vi "Spline Interpolation 1D.vi"(4 "final boundary":T1, 6 "initial boundary":T1, 9 "xi":dbl[](array[numeric]) format="%_6g", 10 "X":dbl[](array[numeric]), 11 "Y":dbl[](array[numeric])) -> (0 "error":i32, 1 "piecewise polynomial":T2 {"x locations" format="%.4g"; "coefficients" format="%.4g"}, 3 "yi":dbl[](array[numeric]) format="%_6g")   [LabVIEW 2017, in "NI_Gmath.lvlib"]
doc: "Performs one-dimensional interpolation using the spline interpolation method based on the lookup table defined by <B>X</B> and <B>Y</B>."
uses:
  <vilib>/gmath/NI_Gmath.lvlib
  <vilib>/gmath/interp.llb/in_piecewise interp poly control.ctl
  <vilib>/Analysis/7linalg.llb/Solve Linear Equations (single right hand).vi
  <vilib>/Analysis/baseanly.llb/Solve Linear Equations By Cholesky.vi
  <vilib>/Analysis/baseanly.llb/Real Matrix to Compact Array.vi
  <vilib>/Analysis/baseanly.llb/Real Compact Tri-Matrix Linear Eqs.vi
  <vilib>/Analysis/7linalg.llb/Solve Linear Eqs (General).vi
  <vilib>/Analysis/7linalg.llb/Solve Linear Eqs (Gen, single right hand).vi
  <vilib>/Analysis/NI_AALPro.lvlib
panel:
  # "Spline Interpolation 1D"
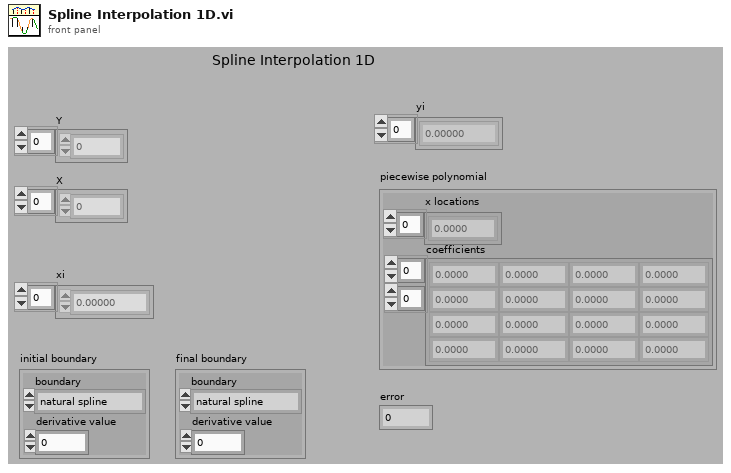
[diagram p1: front panel]
types:
  T1 = cluster{"boundary":enum16{"natural spline", "not-a-knot", "1st derivative", "2nd derivative"}, "derivative value":dbl}
  T2 = typedef "NI_Gmath.lvlib/in_piecewise interp poly control.ctl" = cluster{"x locations":dbl[], "coefficients":dbl[][]}
  T3 = typedef "NI_Matrix.lvlib/RealMatrix.ctl" = dbl[][]
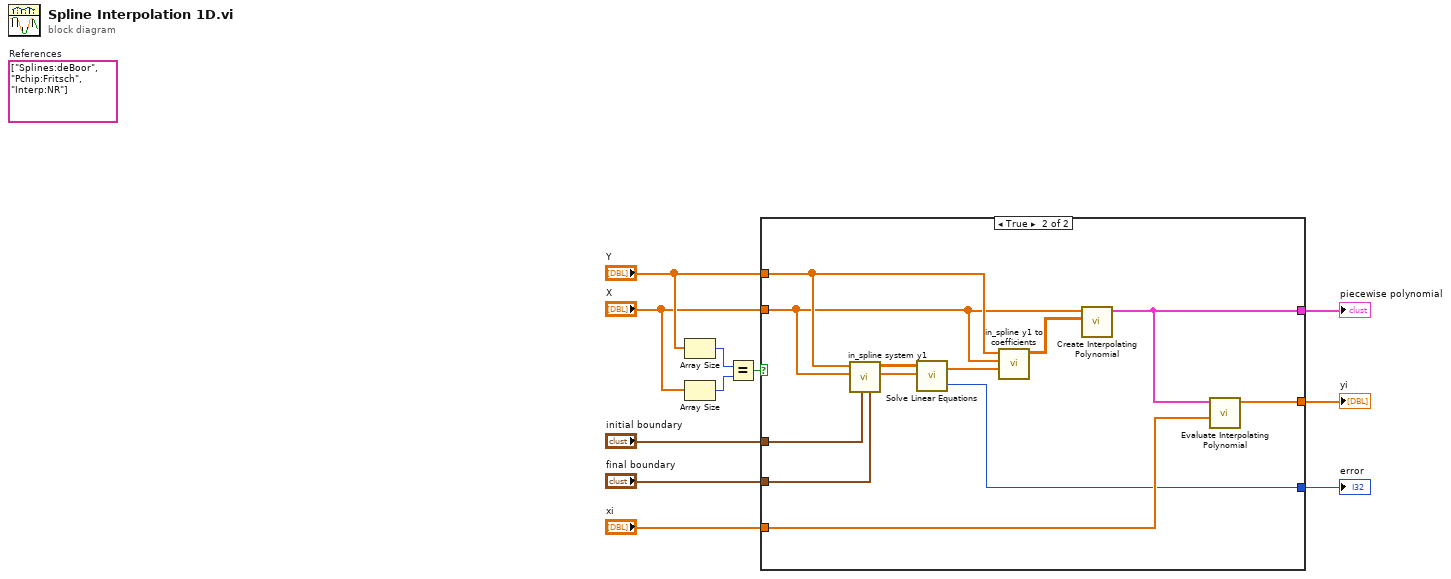
[diagram p0: block diagram]
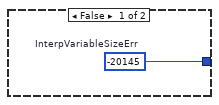
[diagram p2: hidden frame]
diagram:
  (unwired) string[] ["Splines:deBoor", "Pchip:Fritsch", "Interp:NR"]  # References
  n1 = Array Size(array="Y") -> (size(s)=w11:i32)
  n2 = Array Size(array="X") -> (size(s)=w10:i32)
  n3 = Equal?(x=w11, y=w10) -> (x = y?=w7:bool)
  n4 = case shown="True" w7 {
    tunnel: "Y" -> [_ w21]
    tunnel: "X" -> [_ w15]
    tunnel: [w12 w13] -> w6
    tunnel: "initial boundary" -> [_ w20]
    tunnel: "final boundary" -> [_ w19]
    tunnel: "xi" -> [_ w18]
    tunnel: [_ w17] -> w2
    tunnel: [_ w14] -> w1
    frame False {
      w12 = -20145  # InterpVariableSizeErr
    }
    frame True {
      n5 = call <vilib>:"in_spline system y1.vi"("final boundary"=w19, "initial boundary"=w20, "X"=w15, "Y"=w21) -> ("b"=w23:dbl[], "A"=w24:T3)  [unwired: 6 in]
      n6 = call-poly <vilib>:"Solve Linear Equations.vi"("Known Vector"=w23, "Input Matrix"=w24) -> ("error"=w13:i32, "Solution Vector"=w22:dbl[])  [unwired: 1 in]
      n7 = call <vilib>:"in_spline y1 to coefficients.vi"("Y1"=w22, "X"=w15, "Y"=w21) -> ("coefficients"=w16:dbl[][])  [unwired: 8 in]
      n8 = call <vilib>:"Create Interpolating Polynomial.vi"("coefficients"=w16, "x locations"=w15) -> ("piecewise polynomial"=w14:T2)  [unwired: 8 in, 1 out]
      n9 = call <vilib>:"Evaluate Interpolating Polynomial.vi"("xi"=w18, "piecewise polynomial"=w14) -> ("yi"=w17:dbl[])  [unwired: 8 in, 1 out]
    }
  }
  "error" <- w6
  "yi" <- w2
  "piecewise polynomial" <- w1
